vi "Generate INI file path.vi"(1 "VI or App Name":string) -> (0 "appended path":path)   [LabVIEW 2019]
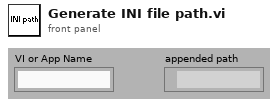
[diagram p1: front panel]
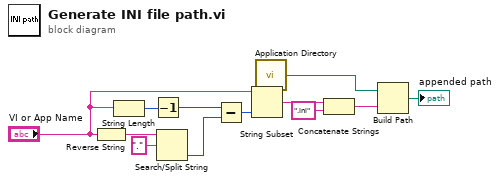
[diagram p0: block diagram]
diagram:
  n1 = Reverse String(1:"VI or App Name") -> (0:w12:string)
  n2 = String Length(string="VI or App Name") -> (length=w9:i32)
  n3 = Decrement(x=w9) -> (x-1=w6:i32)
  n4 = Search/Split String(string=w12, search string/char (-)=".") -> (offset of match=w8:i32)  [unwired: 1 in, 2 out]
  n5 = Subtract(x=w6, y=w8) -> (x-y=w7:i32)
  n6 = String Subset(string="VI or App Name", length (rest)=w7) -> (substring=w5:string)  [unwired: 1 in]
  n7 = call <vilib>:"Application Directory.vi"() -> ("Application Directory"=w2:path)
  n8 = Concatenate Strings(w5, ".ini" ("string")) -> (w3:string)
  n9 = Build Path(base path=w2, name or relative path=w3) -> (appended path=→"appended path":path)
